vi "Runtime Test.vi"() -> ()   [LabVIEW 2015, in "Sequencer Module tests.lvlib"]
doc: "This VI shows an example for how to test the Runtime functionality of the module. This will need to be modified according to module functionality."
uses:
  Sequencer Module tests.lvlib
  module/execution/Sequencer State Cluster.ctl
  module/execution/Sequencer State Enum.ctl
  classes/Step/Execution/StepState.ctl
  classes/Step/Execution/Step Status.ctl
  classes/Step/Execution/Step Flow Control.ctl
  module/execution/Sequencer Control.ctl
  Results.ctl
  Parameters.ctl
  module/execution/Sequencer Module runtime.lvclass
  module/configuration/Sequencer Module configuration.lvclass
  classes/Step/Execution/Step.lvclass
panel:
  out "Steps":i32(listbox)
  out "Sequences":i32(listbox)
  in  "Parameter Values":T1
  out "Cluster":T2
  in  "Sequence Control":T3
  out "State cluster":T4={"Sequencer State"=enum."Start Sequence", "Sequence #"=0, "Active Sequence Name"="", "Active Step"=0, "Step State"={"Step State"=enum."Start", "Flow Control"=enum."Next Step", "Jump Index"=0, "Done"=FALSE}, "Active Step UI Alias"=""}
  out "Channel Names":string[](array[string])
  in  "stop":bool
  out "error":errorcluster
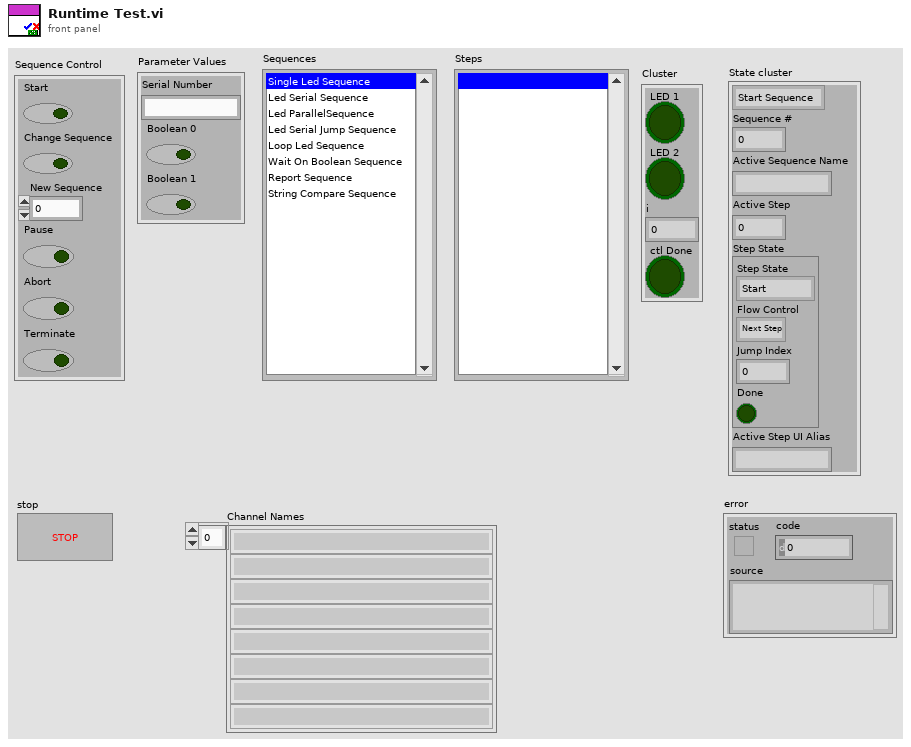
[diagram p1: front panel]
types:
  T1 = typedef "Parameters.ctl" = cluster{"Serial Number":string, "Boolean 0":bool, "Boolean 1":bool}
  T2 = typedef "Sequencer Module tests.lvlib/Results.ctl" = cluster{"LED 1":bool, "LED 2":bool, "i":i32, "ctl Done":bool}
  T3 = typedef "Sequencer Module runtime.lvclass/Sequencer Control.ctl" = cluster{"Start":bool, "Change Sequence":bool, "New Sequence":i32, "Pause":bool, "Abort":bool, "Terminate":bool}
  T4 = typedef "Sequencer Module runtime.lvclass/Sequencer State Cluster.ctl" = cluster{"Sequencer State":T5, "Sequence #":i32, "Active Sequence Name":string, "Active Step":i32, "Step State":T6, "Active Step UI Alias":string}
  T5 = typedef "Sequencer Module runtime.lvclass/Sequencer State Enum.ctl" = enum16{"Idle", "Paused", "Start Sequence", "Run Sequence", "CleanUp Sequence", "Generate Report"}
  T6 = typedef "Step.lvclass/StepState.ctl" = cluster{"Step State":T7, "Flow Control":T8, "Jump Index":i32, "Done":bool}
  T7 = typedef "Step.lvclass/Step Status.ctl" = enum16{"Start", "Passed", "Failed", "Error", "Done", "Terminated", "Skipped", "Running"}
  T8 = typedef "Step.lvclass/Step Flow Control.ctl" = enum16{"Next Step", "Jump"}
  T9 = typedef "TBM channel.lvclass/data tables.ctl" = cluster{"input data":T10, "processing parameter":T10, "processing result":T10, "output data":T10}
  T10 = typedef "tag bus.lvlib/dictionary table pair.ctl" = cluster{"data dictionary":refnum<class "data dictionary.lvclass">, "data table":T11}
  T11 = typedef "tag bus.lvlib/data table.lvlib/data table.ctl" = cluster{"Double":dbl[], "Single":sgl[], "I64":i64[], "I32":i32[], "I16":i16[], "I8":i8[], "U64":u64[], "U32":u32[], "U16":u16[], "U8":u8[], "Boolean":bool[], "String":string[], "Array of Double":cluster{"DBL Array":dbl[]}[], "Array of Single":cluster{"SGL Array":sgl[]}[], "Array of I64":cluster{"I64 Array":i64[]}[], "Array of I32":cluster{"I32 Array":i32[]}[], "Array of I16":cluster{"I16 Array":i16[]}[], "Array of I8":cluster{"I8 Array":i8[]}[], "Array of U64":cluster{"U64 Array":u64[]}[], "Array of U32":cluster{"U32 Array":u32[]}[], "Array of U16":cluster{"U16 Array":u16[]}[], "Array of U8":cluster{"U8 Array":u8[]}[], "Array of Boolean":cluster{"Boolean Array":bool[]}[], "Array of String":cluster{"String Array":string[]}[]}
  T12 = typedef "Parameters Indexes.ctl" = cluster{"Serial Number":i32, "Boolean 0":i32, "Boolean 1":i32}
  T13 = typedef "Sequencer Module tests.lvlib/Results Indexes.ctl" = cluster{"Boolean result 0":i32, "Boolean result 1":i32, "i":i32, "Complete":i32}
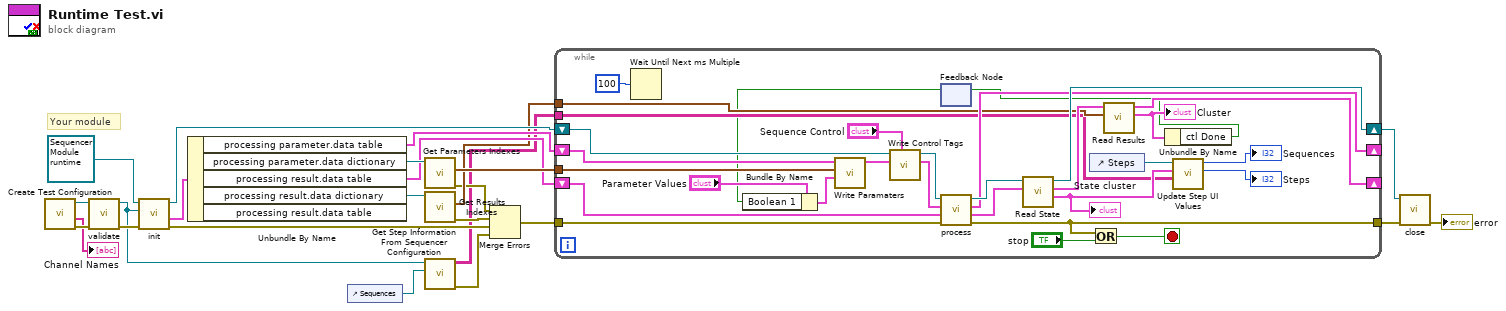
[diagram p0: block diagram]
diagram:
  # "Your module"
  n1 = call "Create Test Configuration.vi"() -> ("error out"=w22:errorcluster, "Channel Names"=→"Channel Names":string[], "Module Configuration"=w12:refnum<class "Sequencer Module configuration.lvclass">)  [unwired: 6 in, 3 out]
  n2 = call-dynamic "validate.vi"("error in"=w22, "Sequencer Module configuration in"=w12) -> ("error out"=w23:errorcluster, "Sequencer Module configuration out"=w4:refnum<class "Sequencer Module configuration.lvclass">)  [unwired: 8 in]
  n3 = call-dynamic "init.vi"("error in"=w23, "TBM module configuration in"=w4, "Sequencer Module runtime in"=refnum<class "Sequencer Module runtime.lvclass"> refnum ("tag bus configurable plugin module")) -> ("error out"=w6:errorcluster, "data allocations"=w18:T9, "Sequencer Module runtime out"=w19:refnum<class "Sequencer Module runtime.lvclass">)  [unwired: 5 in, 1 out]
  n4 = Unbundle By Name(w18) -> ("processing parameter.data table"=w11:T11, "processing parameter.data dictionary"=w21:refnum<class "data dictionary.lvclass">, "processing result.data table"=w10:T11, "processing result.data dictionary"=w14:refnum<class "data dictionary.lvclass">)  [unwired: 1 out]
  n5 = control-ref of="Sequences"() -> (w1:refnum<vi>)
  n6 = call "Get Parameters Indexes.vi"("data dictionary in"=w21) -> ("error out"=w5:errorcluster, "Parameter Indexes"=w15:T12)  [unwired: 9 in]
  n7 = call "Get Results Indexes.vi"("data dictionary in"=w14) -> ("error out"=w9:errorcluster, "Results Indexes"=w8:T13)  [unwired: 9 in]
  n8 = call "Get Step Information From Sequencer Configuration.vi"("LstBox Refnum"=w1, "Sequencer Module configuration in"=w4) -> ("error out"=w3:errorcluster, "Array"=w2:string[][])  [unwired: 8 in]
  n9 = Merge Errors(w5, w9, w6, w3) -> (w7:errorcluster)
  n10 = while {
    tunnel: w15 -> [w36]
    shift-right: [w46] -> w17
    shift-left: w19 -> [w43]
    shift-right: [w38] -> _
    shift-left: w10 -> [w54]
    shift-right: [w44] -> _
    shift-left: w11 -> [w35]
    tunnel: w8 -> [w39]
    tunnel: w7 -> [w53]
    tunnel: [w49] -> w16
    tunnel: w2 -> [w32]
    stop <- w50 stop-if-true
    n11 = Wait Until Next ms Multiple(millisecond multiple=u32 100) -> ()  [unwired: 1 out]
    n12 = feedback #1() -> (w25:bool)  [unwired: 1 in]
    n13 = Bundle By Name(cluster="Parameter Values", "Boolean 1"=w25) -> (w28:T1)
    n14 = call "Write Paramaters.vi"("Parameter Values"=w28, "Parameter Indexes"=w36, "data table in"=w35) -> ("data table out"=w37:T11)  [unwired: 7 in, 1 out]
    n15 = call "Write Control Tags.vi"("Sequence Control"="Sequence Control", "Prameter allocation in"=w37, "Sequencer Module runtime in"=w43) -> ("Parameter allocation out"=w41:T11, "Sequencer Module runtime out"=w42:refnum<class "Sequencer Module runtime.lvclass">)  [unwired: 7 in]
    n16 = call-dynamic "process.vi"("error in"=w53, "result allocation"=w54, "parameters"=w41, "module in"=w42) -> ("error out"=w49:errorcluster, "results"=w47:T11, "parameter allocation"=w44:T11, "module out"=w48:refnum<class "Sequencer Module runtime.lvclass">)  [unwired: 4 in]
    n17 = call "Read State.vi"("result allocation in"=w47, "Sequencer Module runtime in"=w48) -> ("State cluster"=w33:T4, "result allocation out"=w45:T11, "Sequencer Module runtime out"=w46:refnum<class "Sequencer Module runtime.lvclass">)  [unwired: 7 in]
    "State cluster" <- w33
    n18 = control-ref of="Steps"() -> (w29:refnum<vi>)
    n19 = Or(x=w49, y="stop") -> (x .or. y?=w50:bool)
    n20 = call "Read Results.vi"("Results Indexes"=w39, "result allocation in"=w45) -> ("Cluster"=w27:T2, "data table out"=w38:T11)  [unwired: 8 in]
    "Cluster" <- w27
    n21 = Unbundle By Name(w27) -> ("ctl Done"=w26:bool)
    n22 = feedback-in #1(w26) -> ()
    n23 = call "Update Step UI Values.vi"("Array"=w32, "State cluster"=w33, "ListBox in"=w29) -> ("index of element"=→"Steps":i32, "Sequence #"=→"Sequences":i32)  [unwired: 7 in]
  }
  n24 = call-dynamic "close.vi"("error in"=w16, "Sequencer Module runtime in"=w17) -> ("error out"=→"error":errorcluster)  [unwired: 9 in]
